vi "Automatic Image Scale V2.vi"(0 "Document":refnum<k24>, 1 "Y offset (point)":sgl, 2 "Scale Type":T1, 5 "GetInstanceImage IN":refnum<k24>, 9 "Scale percent IN":sgl, 11 "error in (no error)":errorcluster, 12 "Box":cluster{"width":sgl, "height":sgl}, 14 "Rotate?":bool) -> (3 "Scaled Image width":sgl, 4 "Document duplicate":refnum<k24>, 6 "GetInstanceImage OUT":refnum<k24>, 10 "Scale percent OUT":sgl, 15 "error out":errorcluster)   [LabVIEW 2019]
doc: "Version 2.0\nDeveloped by Jean-Marc Simard\nCopyright © 2012, Exaprom Inc.\nAll rights reserved.\nLicense: BSD\n\nWith iTextSharp 4.1.6 (http://itextsharp.sourceforge.net)\nunder Mozilla Public License Version 1.1\n(http://www.mozilla.org/MPL/MPL-1.1.html)"
uses:
  C:/Program Files/National Instruments/LabVIEW 2019/user.lib/Exaprom PDF/DLL/itextsharp.dll
  DLL/itextsharp.dll
  <userlib>/Exaprom PDF/Controls/Image Controls/Image Scale Type.ctl
  <userlib>/Exaprom PDF/LV Class/PDF Report Class/PDF Report Class.lvclass
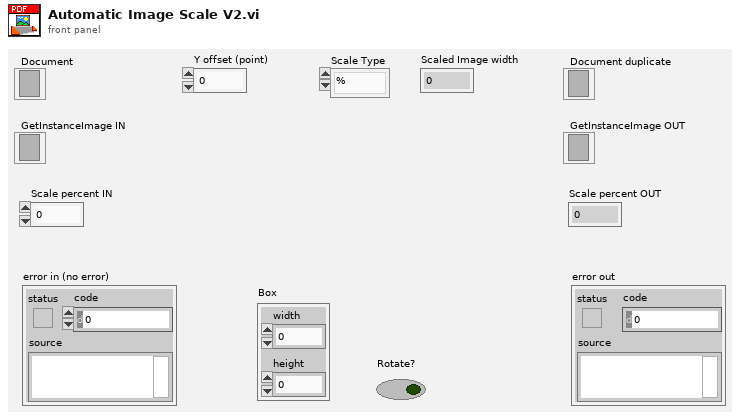
[diagram p1: front panel]
types:
  T1 = typedef "Image Scale Type.ctl" = enum16{"%", "Height", "Width"}
  T2 = typedef "Page dimensions.ctl" = cluster{"Start at page":i32, "Page Size":T3, "Orientation":T4, "widht":sgl, "height":sgl, "Margin left":sgl, "Margin right":sgl, "Margin top":sgl, "Margin bottom":sgl, "X0":sgl, "X1":sgl, "Y0":sgl, "Y1":sgl}
  T3 = typedef "Page size.ctl" = i32
  T4 = typedef "Page Orientation.ctl" = enum16{"Portrait", "Landscape"}
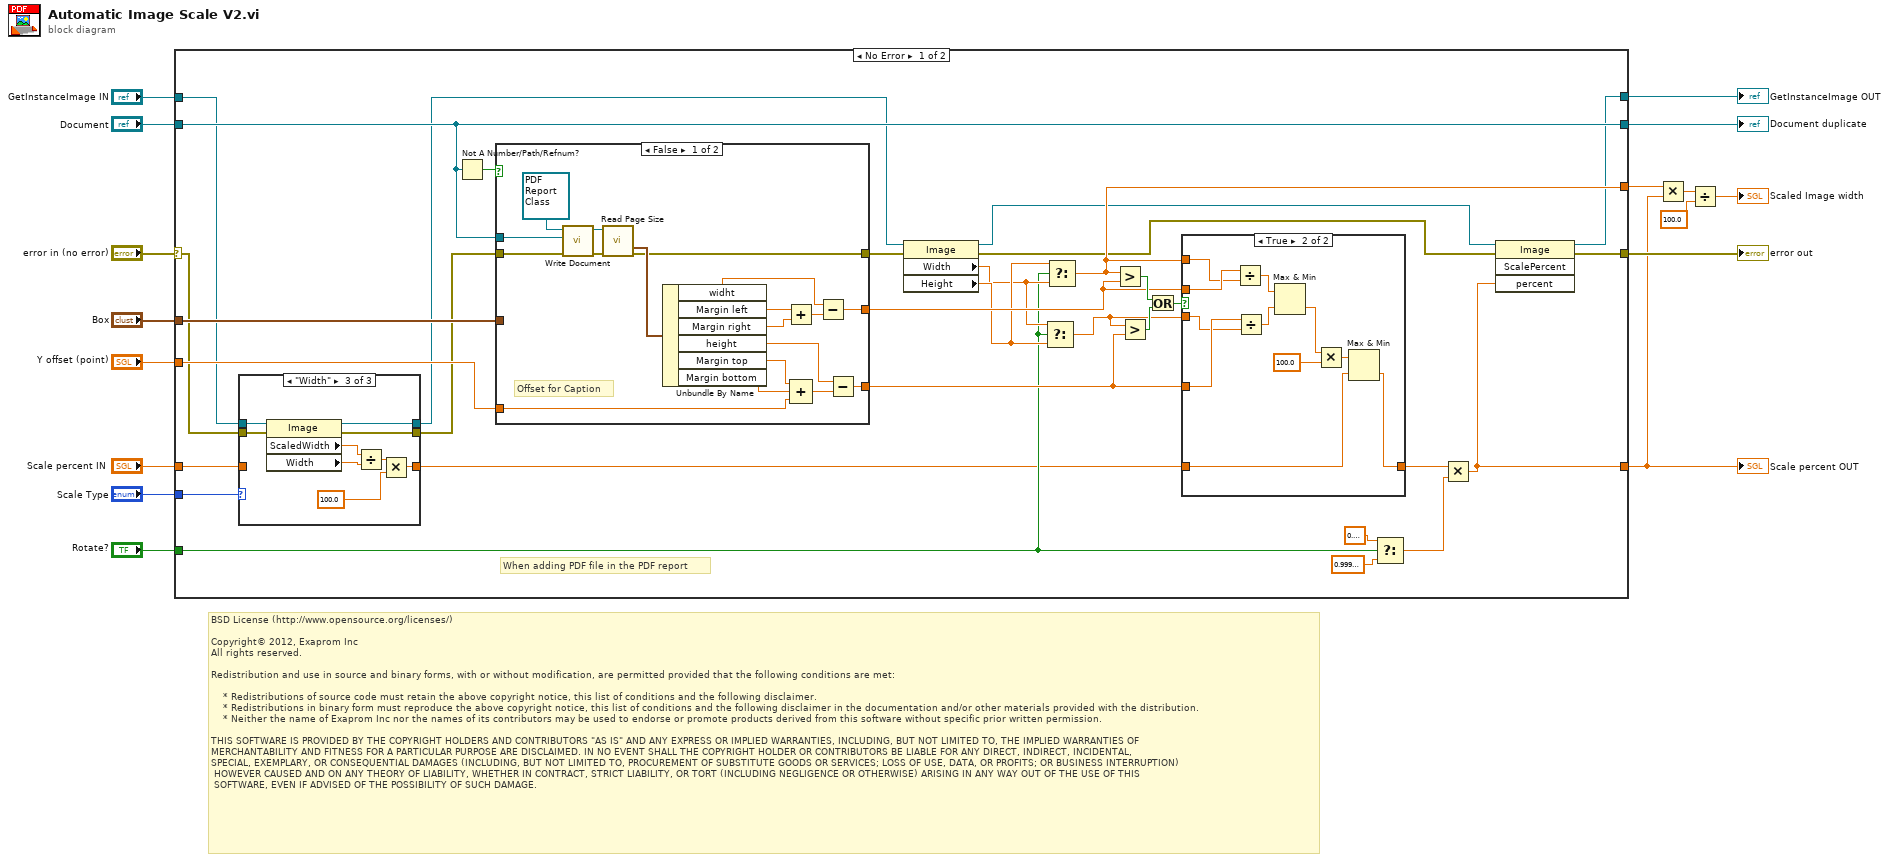
[diagram p0: block diagram]
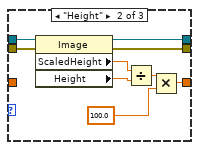
[diagram p3: hidden frame]
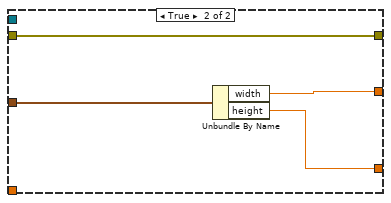
[diagram p4: hidden frame]
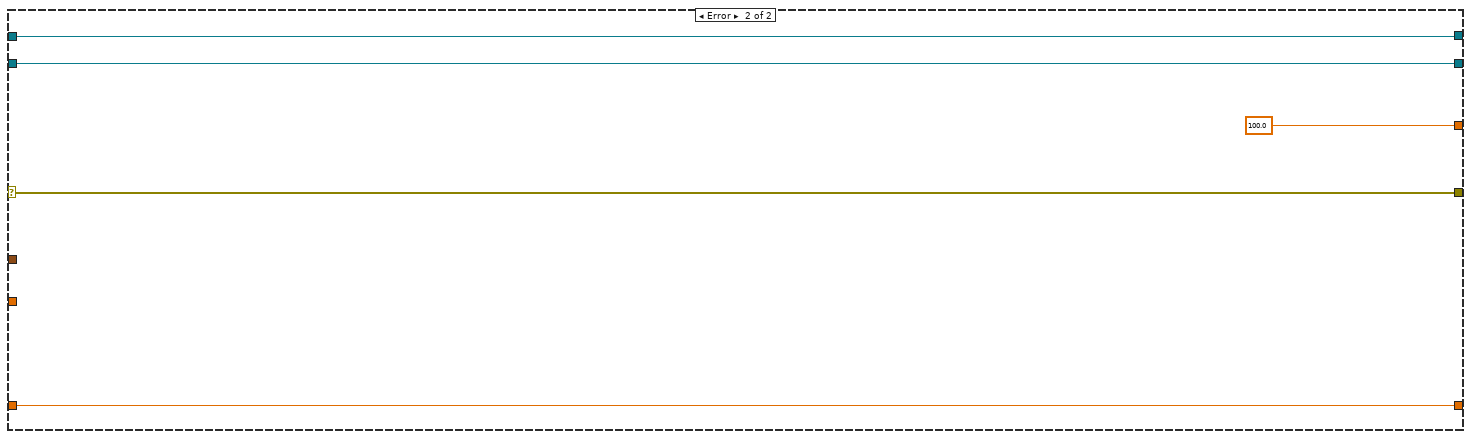
[diagram p6: hidden frame]
diagram:
  # "BSD License (http://www.opensource.org/licenses/)\n\nCopyright© 2012, Exaprom Inc\nAll rights reserved.\n\nRedistribution and use in source and binary forms, with or without modification, are permitted provided that the following conditions are met:\n\n    * Redistributions of source code must retain the above copyright notice, this list of conditions and the following disclaimer.\n    * Redistributions in binary form must reproduce the above copyright notice, this list of conditions and the following disclaimer in the documentation and/or other materials provided with the distribution.\n    * Neither the name of Exaprom Inc nor the names of its contributors may be used to endorse or promote products derived from this software without specific prior written permission.\n\nTHIS SOFTWARE IS PROVIDED BY THE COPYRIGHT HOLDERS AND CONTRIBUTORS \"AS IS\" AND ANY EXPRESS OR IMPLIED WARRANTIES, INCLUDING, BUT NOT LIMITED TO, THE IMPLIED WARRANTIES OF \nMERCHANTABILITY AND FITNESS FOR A PARTICULAR PURPOSE ARE DISCLAIMED. IN NO EVENT SHALL THE COPYRIGHT HOLDER OR CONTRIBUTORS BE LIABLE FOR ANY DIRECT, INDIRECT, INCIDENTAL,\nSPECIAL, EXEMPLARY, OR CONSEQUENTIAL DAMAGES (INCLUDING, BUT NOT LIMITED TO, PROCUREMENT OF SUBSTITUTE GOODS OR SERVICES; LOSS OF USE, DATA, OR PROFITS; OR BUSINESS INTERRUPTION)\n HOWEVER CAUSED AND ON ANY THEORY OF LIABILITY, WHETHER IN CONTRACT, STRICT LIABILITY, OR TORT (INCLUDING NEGLIGENCE OR OTHERWISE) ARISING IN ANY WAY OUT OF THE USE OF THIS\n SOFTWARE, EVEN IF ADVISED OF THE POSSIBILITY OF SUCH DAMAGE."
  n1 = case shown="No Error" "error in (no error)" {
    selector: "error in (no error)" -> [w20 w105]
    tunnel: "GetInstanceImage IN" -> [w18 w107]
    tunnel: "Scale percent IN" -> [w21 w104]
    tunnel: [w26 w104] -> w7
    tunnel: [w40 w106] -> w14
    tunnel: [w24 w107] -> w13
    tunnel: "Document" -> [w40 w106]
    tunnel: [w28 w105] -> w11
    tunnel: "Box" -> [w41 _]
    tunnel: [w36 sgl 100.0 ("Width")] -> w8
    tunnel: "Y offset (point)" -> [w38 _]
    tunnel: "Rotate?" -> [w29 _]
    tunnel: "Scale Type" -> [w23 _]
    frame No Error {
      # "When adding PDF file in the PDF report"
      n2 = case shown="\"Width\"" w23 {
        tunnel: [w50 w55 w64] -> w22
        tunnel: w21 -> [w50 _ _]
        tunnel: w20 -> [w49 w54 w63]
        tunnel: [w49 w53 w62] -> w19
        tunnel: [w48 w52 w61] -> w17
        tunnel: w18 -> [w48 w51 w60]
        frame "%", Default {
        }
        frame "Height" {
          n3 = property class="Image"(reference=w51, error in=w54) -> (reference out=w52:refnum<k24>, error out=w53:errorcluster, "ScaledHeight"=w57:sgl, "Height"=w56:sgl)
          n4 = Divide(x=w57, y=w56) -> (x/y=w58:sgl)
          n5 = Multiply(x=w58, y=sgl 100.0) -> (x*y=w55:sgl)
        }
        frame "Width" {
          n6 = property class="Image"(reference=w60, error in=w63) -> (reference out=w61:refnum<k24>, error out=w62:errorcluster, "ScaledWidth"=w66:sgl, "Width"=w65:sgl)
          n7 = Divide(x=w66, y=w65) -> (x/y=w67:sgl)
          n8 = Multiply(x=w67, y=sgl 100.0) -> (x*y=w64:sgl)
        }
      }
      n9 = Not A Number/Path/Refnum?(number/path/refnum=w40) -> (NaN/Path/Refnum?=w42:bool)
      n10 = case shown="False" w42 {
        tunnel: w40 -> [w70 _]
        tunnel: [w74 w90] -> w47
        tunnel: [w84 w88] -> w44
        tunnel: [w83 w87] -> w39
        tunnel: w19 -> [w82 w90]
        tunnel: w41 -> [_ w89]
        tunnel: w38 -> [w73 _]
        frame False {
          # "Offset for Caption"
          n11 = call-dynamic "Write Document.vi"("error in (no error)"=w82, "Document"=w70, "PDF Report Class in"=refnum<class "PDF Report Class.lvclass"> refnum ("PDF Report")) -> ("error out"=w72:errorcluster, "PDF Report Class out"=w69:refnum<class "PDF Report Class.lvclass">)  [unwired: 7 in]
          n12 = call <userlib>:"Read Page Size.vi"("PDF Report"=w69, "error in (no error)"=w72) -> ("Page (points)"=w81:T2, "error out"=w74:errorcluster)  [unwired: 12 out]
          n13 = Unbundle By Name(w81) -> ("widht"=w75:sgl, "Margin left"=w76:sgl, "Margin right"=w77:sgl, "height"=w78:sgl, "Margin top"=w80:sgl, "Margin bottom"=w79:sgl)
          n14 = Add(x=w76, y=w77) -> (x+y=w86:sgl)
          n15 = Compound Arithmetic op=ADD(w80, w79, w73) -> (w85:sgl)
          n16 = Subtract(x=w75, y=w86) -> (x-y=w84:sgl)
          n17 = Subtract(x=w78, y=w85) -> (x-y=w83:sgl)
        }
        frame True {
          n18 = Unbundle By Name(w89) -> ("width"=w88:sgl, "height"=w87:sgl)
        }
      }
      n19 = property class="Image"(reference=w17, error in=w47) -> (reference out=w25:refnum<k24>, error out=w27:errorcluster, "Width"=w33:sgl, "Height"=w34:sgl)
      n20 = Select(t=w33, s=w29, f=w34) -> (s? t:f=w35:sgl)
      n21 = Select(t=w34, s=w29, f=w33) -> (s? t:f=w36:sgl)
      n22 = Greater?(x=w36, y=w44) -> (0:w45:bool)
      n23 = Greater?(x=w35, y=w39) -> (0:w46:bool)
      n24 = Or(x=w45, y=w46) -> (x .or. y?=w43:bool)
      n25 = case shown="True" w43 {
        tunnel: w36 -> [_ w101]
        tunnel: w44 -> [_ w102]
        tunnel: w35 -> [_ w99]
        tunnel: w39 -> [_ w100]
        tunnel: w22 -> [w91 w96]
        tunnel: [w91 w95] -> w37
        frame False {
        }
        frame True {
          n26 = Divide(x=w102, y=w101) -> (x/y=w98:sgl)
          n27 = Divide(x=w100, y=w99) -> (x/y=w97:sgl)
          n28 = Max & Min(x=w98, y=w97) -> (min(x,y)=w93:sgl)  [unwired: 1 out]
          n29 = Multiply(x=w93, y=sgl 100.0) -> (x*y=w94:sgl)
          n30 = Max & Min(x=w94, y=w96) -> (min(x,y)=w95:sgl)  [unwired: 1 out]
        }
      }
      n31 = Select(t=sgl 0.9 ("y"), s=w29, f=sgl 0.999 ("y")) -> (s? t:f=w30:sgl)
      n32 = Multiply(x=w37, y=w30) -> (x*y=w26:sgl)
      n33 = invoke class="Image" method="ScalePercent"(reference=w25, error in=w27, "percent"=w26) -> (reference out=w24:refnum<k24>, error out=w28:errorcluster)  [unwired: 1 in, 2 out]
    }
    frame Error {
    }
  }
  "Scale percent OUT" <- w7
  "Document duplicate" <- w14
  "GetInstanceImage OUT" <- w13
  "error out" <- w11
  n34 = Multiply(x=w8, y=w7) -> (x*y=w6:sgl)
  n35 = Divide(x=w6, y=sgl 100.0) -> (x/y=→"Scaled Image width":sgl)
